vi "TestUntitled 1.vi"() -> ()   [LabVIEW 2020]
uses:
  <vilib>/userDefined/High Color/IMAQdx.ctl
panel:
  out "Status":bool
  out "Detected sign":string
  out "Python Error Out":errorcluster
  in  "Off/On":bool caption="Start/Stop Vision"
  out "error out 4":errorcluster
  out "Live view":T1(plugin-control)
  out "Camera Status":errorcluster
  in  "Exit program":bool
  out "IMAQ Err":errorcluster
  in  "Camera Device":T2="cam0"
  # "Vision control panel"
  # "Camera configuration"
  # "Error section"
  # "Tymczasowe"
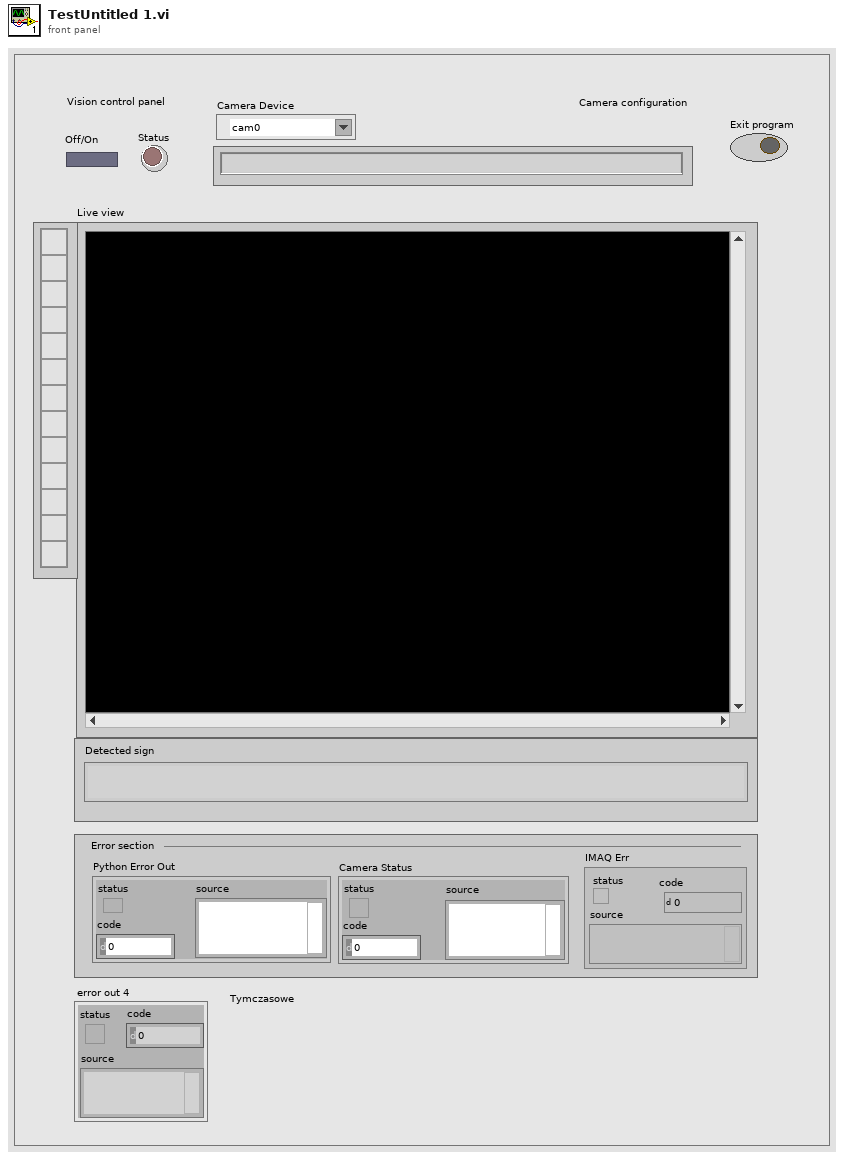
[diagram p1: front panel]
types:
  T1 = typedef "IMAQ Image.ctl" = refnum<image>
  T2 = typedef "IMAQdx.ctl" = refnum<k21>
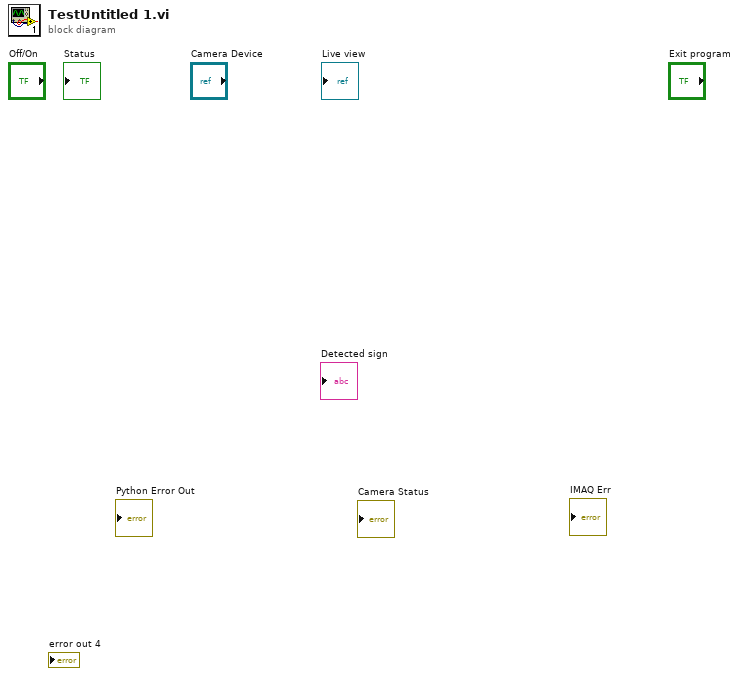
[diagram p0: block diagram]
diagram:
